vi "PH_BlackBox.PC Move in.vi"(0 "i ref in":refnum<vi>, 2 "Move in?":bool, 5 "error in (no error)":errorcluster) -> (14 "i ref out":refnum<vi>, 19 "error out":errorcluster)   [LabVIEW 2014, in "PH_BlackBox.lvlib"]
doc: "This is the action done in the event case \"SetDirection\"."
uses:
  PH_BlackBox.lvlib
  PH_StatusHandler/PH_StatusHandler.Status.ctl
  PH_Common/PH_Common.lvlib
  PH_Beckhoff_Common/PH_Beckhoff_Common.lvlib
  PH_StatusHandler/PH_StatusHandler.lvlib
  PH_Beckhoff/PH_Beckhoff.lvlib
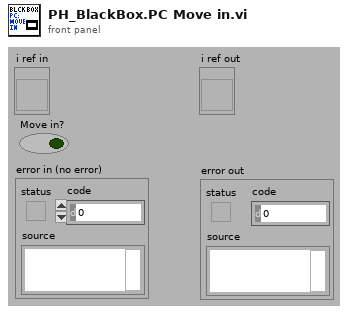
[diagram p1: front panel]
types:
  T1 = typedef "PH_StatusHandler.lvlib/PH_StatusHandler.Status.ctl" = i16
  T2 = typedef "PH_BlackBox.lvlib/PH_BlackBox.i attribute.ctl" = cluster{"BB Remote Controlled?":bool, "GUI Refs":T3, "Position IN":T1, "Position OUT":T1, "BB Remote Controlled by other Instance?":bool, "Recipient":string, "Number":i32, "Caption Move":string, "Caption Out":string, "Caption In":string}
  T3 = typedef "PH_BlackBox.lvlib/PH_BlackBox.GUI Refs.ctl" = cluster{"MOVE IN":refnum<vi>, "MOVE":refnum<vi>, "IN":refnum<vi>, "OUT":refnum<vi>, "REMOTE":refnum<vi>, "GUI-Knob Move":refnum<vi>, "GUI-Knob Move in":refnum<vi>, "POWER ON":refnum<vi>, "Delete":refnum<vi>, "Function Textfield":refnum<vi>}
  T4 = typedef "PH_Beckhoff_Common.lvlib/PH_Beckhoff_Common.BB Tagnames.ctl" = cluster{"Sensor Remote controlled":string, "Sensor Out":string, "Sensor In":string, "Actor Direction In":string, "Actor Move":string, "Sensor Power ok":string, "Instance":string}
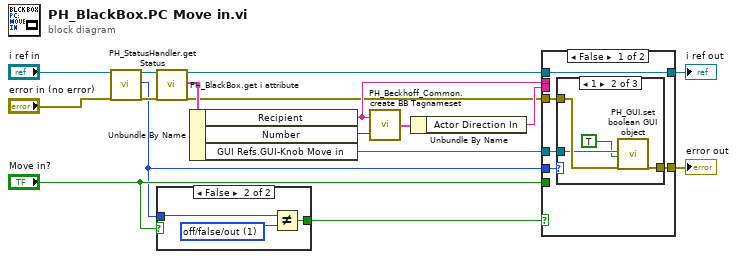
[diagram p0: block diagram]
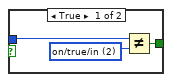
[diagram p2: hidden frame]
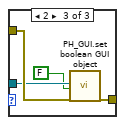
[diagram p4: hidden frame]
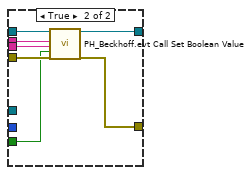
[diagram p5: hidden frame]
diagram:
  n1 = call "PH_StatusHandler.get Status.vi"("VI in"="i ref in", "error in"="error in (no error)") -> ("VI out"=w2:refnum<vi>, "Status"=w1:T1, "error out"=w4:errorcluster)  [unwired: 15 in]
  n2 = call "PH_BlackBox.get i attribute.vi"("i ref in"=w2, "error in (no error)"=w4) -> ("i ref out"=w6:refnum<vi>, "i attribute"=w15:T2, "error out"=w5:errorcluster)  [unwired: 15 in]
  n3 = case shown="False" "Move in?" {
    tunnel: w1 -> [w20 w23]
    tunnel: [w19 w22] -> w11
    frame True {
      w18 = T1 2 items=["no info", "off/false/out", "on/true/in", "Failure", "Alarm", "Status 1", "Status 2", "Status 3"] ("Status")
      n4 = Not Equal?(x=w20, y=w18) -> (x != y?=w19:bool)
    }
    frame False {
      w21 = T1 1 items=["no info", "off/false/out", "on/true/in", "Failure", "Alarm", "Status 1", "Status 2", "Status 3"] ("Status")
      n5 = Not Equal?(x=w23, y=w21) -> (x != y?=w22:bool)
    }
  }
  n6 = Unbundle By Name(w15) -> ("Recipient"=w10:string, "Number"=w9:i32, "GUI Refs.GUI-Knob Move in"=w16:refnum<vi>)
  n7 = call "PH_Beckhoff_Common.create BB Tagnameset.vi"("#"=w9, "Instance Name"=w10) -> ("output cluster"=w8:T4)
  n8 = Unbundle By Name(w8) -> ("Actor Direction In"=w7:string)
  n9 = case shown="False" w11 {
    tunnel: [w28 w42] -> w12
    tunnel: [w26 w41] -> w13
    tunnel: w10 -> [_ w40]
    tunnel: w6 -> [w28 w44]
    tunnel: w5 -> [w27 w43]
    tunnel: w16 -> [w25 _]
    tunnel: w1 -> [w24 _]
    tunnel: w7 -> [_ w39]
    tunnel: "Move in?" -> [_ w38]
    frame False {
      n10 = case shown="1" w24 {
        tunnel: w27 -> [w29 w33 w37]
        tunnel: [w29 w32 w36] -> w26
        tunnel: w25 -> [_ w31 w35]
        frame 0, Default {
        }
        frame 1 {
          n11 = call "PH_GUI.set boolean GUI object.vi"("Boolean Knob GUI Ref"=w31, "Value"=TRUE, "error in (no error)"=w33) -> ("error out"=w32:errorcluster)  [unwired: 16 in]
        }
        frame 2 {
          n12 = call "PH_GUI.set boolean GUI object.vi"("Boolean Knob GUI Ref"=w35, "Value"=FALSE, "error in (no error)"=w37) -> ("error out"=w36:errorcluster)  [unwired: 16 in]
        }
      }
    }
    frame True {
      n13 = call "PH_Beckhoff.evt Call Set Boolean Value.vi"("i ref in"=w44, "Beckhoff Instance"=w40, "Tagname to set"=w39, "Value"=w38, "error in"=w43) -> ("i ref out"=w42:refnum<vi>, "error out"=w41:errorcluster)  [unwired: 13 in]
    }
  }
  "error out" <- w13
  "i ref out" <- w12
